vi "Protocol.Parse Message Type.vi"(0 "CAN frame":T1 {"payload" format="%x"; "timestamp" format="%<%.7X\n%x>T"; "type" items=["CAN Data"=0, "CAN Remote"=1, "CAN Bus Error"=2, "CAN 2.0 Data"=8, "CAN FD Data"=16, "CAN FD+BRS Data"=24, "J1939 Data"=192, "Delay"=224, "Log Trigger"=225, "Start Trigger"=226]; "identifier" format="%x"}, 11 "error in":errorcluster) -> (4 "CAN frame":T1 {"payload" format="%x"; "timestamp" format="%<%.7X\n%x>T"; "type" items=["CAN Data"=0, "CAN Remote"=1, "CAN Bus Error"=2, "CAN 2.0 Data"=8, "CAN FD Data"=16, "CAN FD+BRS Data"=24, "J1939 Data"=192, "Delay"=224, "Log Trigger"=225, "Start Trigger"=226]; "identifier" format="%x"}, 6 "State":T3=enum."ACL", 8 "PDU F":u8 format="%.0x", 10 "PDU S":u8, 15 "error out":errorcluster)   [LabVIEW 2015, in "J1939 Addon Engine.lvlib"]
uses:
  J1939 Addon Engine.lvlib
  Shared/J1939 Utilities/Types/Message Types.ctl
  <vilib>/xnet/xnet.llb/XNET Frame CAN.ctl
  <vilib>/xnet/xnet.llb/XNET Frame Type CAN.ctl
  Shared/J1939 Utilities/J1939 Utilities.lvlib
panel:
  # "238"
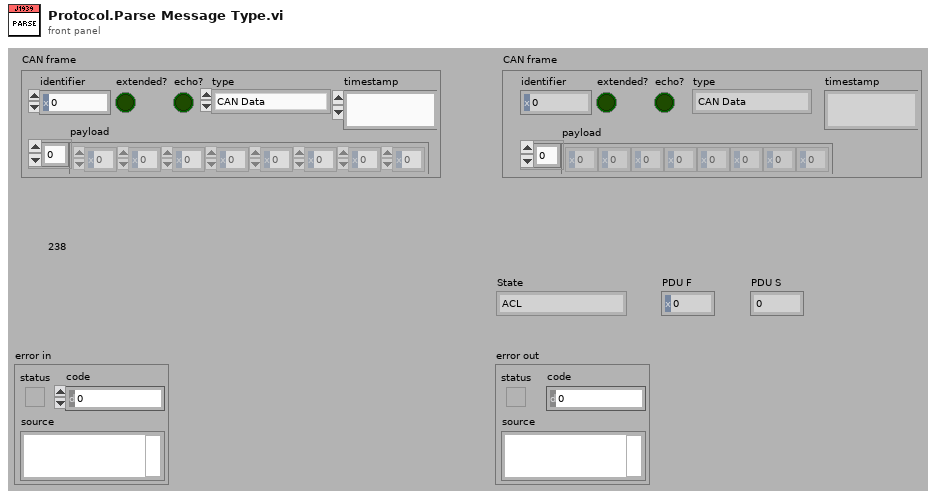
[diagram p1: front panel]
types:
  T1 = typedef "XNET Frame CAN.ctl" = cluster{"timestamp":timestamp, "payload":u8[], "identifier":u32, "type":T2, "extended?":bool, "echo?":bool}
  T2 = typedef "XNET Frame Type CAN.ctl" = u8
  T3 = typedef "J1939 Addon Shared.lvlib/J1939 Utilities.lvlib/Message Types.ctl" = enum8{"PDU 1", "RQST2", "XFER", "ACKM", "RQST", "TP.DT - RTS/CTS", "TP.DT - BAM", "TP.CM - RTS", "TP.CM - CTS", "TP.CM - EndofMsgACK", "TP.CM - BAM", "TP.CM - Abort", "TP.CM - Error", "ACL", "Proprietary A", "PDU 2", "Proprietary B", "Error"}
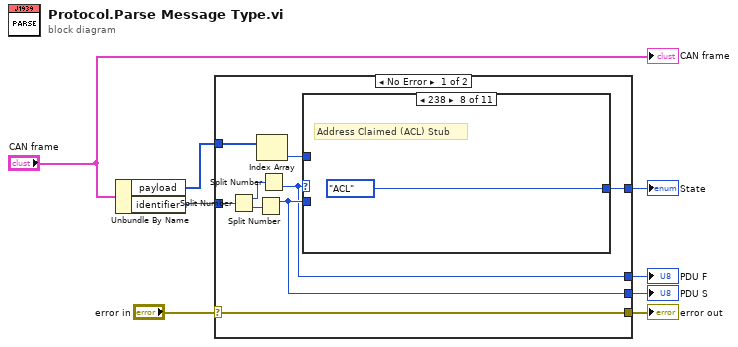
[diagram p0: block diagram]
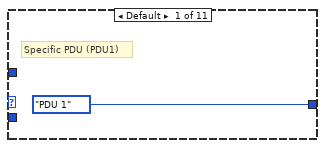
[diagram p2: hidden frame]
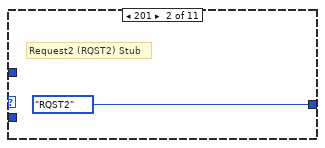
[diagram p3: hidden frame]
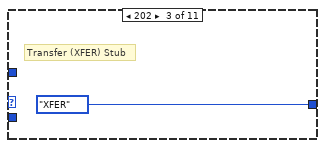
[diagram p4: hidden frame]
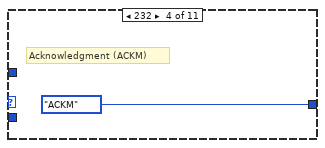
[diagram p5: hidden frame]
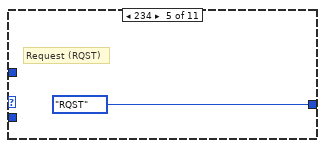
[diagram p6: hidden frame]
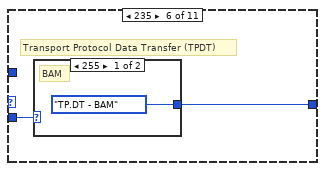
[diagram p7: hidden frame]
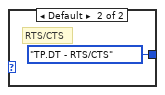
[diagram p8: hidden frame]
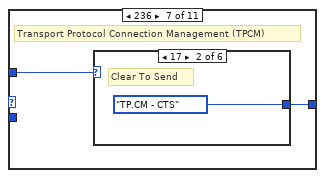
[diagram p9: hidden frame]
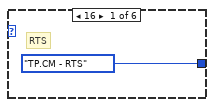
[diagram p10: hidden frame]
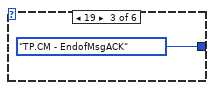
[diagram p11: hidden frame]
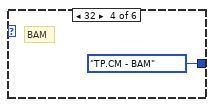
[diagram p12: hidden frame]
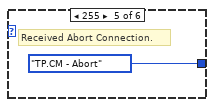
[diagram p13: hidden frame]
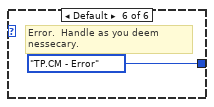
[diagram p14: hidden frame]
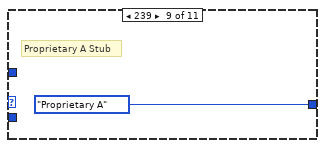
[diagram p15: hidden frame]
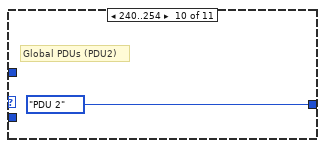
[diagram p16: hidden frame]
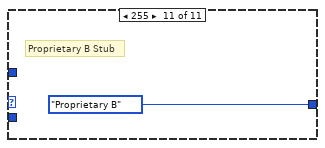
[diagram p17: hidden frame]
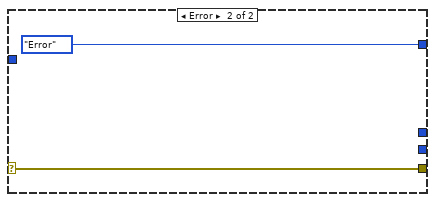
[diagram p18: hidden frame]
diagram:
  n1 = Unbundle By Name("CAN frame") -> ("payload"=w4:u8[], "identifier"=w5:u32)
  n2 = case shown="No Error" "error in" {
    selector: "error in" -> [w15 w40]
    tunnel: w4 -> [w17 _]
    tunnel: w5 -> [w11 _]
    tunnel: [w15 w40] -> w7
    tunnel: [w14 Message_Types."Error" ("State")] -> w6
    tunnel: [w10 _] -> w3
    tunnel: [w9 _] -> w2
    frame No Error {
      n3 = Split Number(x=w11) -> (hi(x)=w13:u16, lo(x)=w12:u16)
      n4 = Split Number(x=w12) -> (hi(x)=w10:u8)  [unwired: 1 out]
      n5 = Index Array(array=w17) -> (element=w16:u8)  [unwired: 1 in]
      n6 = Split Number(x=w13) -> (lo(x)=w9:u8)  [unwired: 1 out]
      n7 = case shown="238" w9 {
        tunnel: w10 -> [_ _ _ _ _ w24 _ _ _ _ _]
        tunnel: w16 -> [_ _ _ _ _ _ w27 _ _ _ _]
        tunnel: [Message_Types."PDU 1" ("State") Message_Types."RQST2" ("State") Message_Types."XFER" ("State") Message_Types."ACKM" ("State") Message_Types."RQST" ("State") w23 w28 Message_Types."ACL" ("State") Message_Types."Proprietary A" ("State") Message_Types."PDU 2" ("State") Message_Types."Proprietary B" ("State")] -> w14
        frame Default {
          # "Specific PDU (PDU1)"
        }
        frame 201 {
          # "Request2 (RQST2) Stub"
        }
        frame 202 {
          # "Transfer (XFER) Stub"
        }
        frame 232 {
          # "Acknowledgment (ACKM)"
        }
        frame 234 {
          # "Request (RQST)"
        }
        frame 235 {
          # "Transport Protocol Data Transfer (TPDT)"
          n8 = case shown="255" w24 {
            tunnel: [Message_Types."TP.DT - BAM" ("State") Message_Types."TP.DT - RTS/CTS" ("State")] -> w23
            frame 255 {
              # "BAM"
            }
            frame Default {
              # "RTS/CTS"
            }
          }
        }
        frame 236 {
          # "Transport Protocol Connection Management (TPCM)"
          n9 = case shown="17" w27 {
            tunnel: [Message_Types."TP.CM - RTS" ("State") Message_Types."TP.CM - CTS" ("State") Message_Types."TP.CM - EndofMsgACK" ("State") Message_Types."TP.CM - BAM" ("State") Message_Types."TP.CM - Abort" ("State") Message_Types."TP.CM - Error" ("State")] -> w28
            frame 16 {
              # "RTS"
            }
            frame 17 {
              # "Clear To Send"
            }
            frame 19 {
            }
            frame 32 {
              # "BAM"
            }
            frame 255 {
              # "Received Abort Connection."
            }
            frame Default {
              # "Error.  Handle as you deem nessecary."
            }
          }
        }
        frame 238 {
          # "Address Claimed (ACL) Stub"
        }
        frame 239 {
          # "Proprietary A Stub"
        }
        frame 240..254 {
          # "Global PDUs (PDU2)"
        }
        frame 255 {
          # "Proprietary B Stub"
        }
      }
    }
    frame Error {
    }
  }
  "error out" <- w7
  "State" <- w6
  "PDU S" <- w3
  "PDU F" <- w2
  "CAN frame" <- "CAN frame"
